vi "GreyRings.vi"(8 "error in (no error)":errorcluster, 11 "MAUI in":refnum<class "MAUI.lvclass">) -> (0 "error out":errorcluster, 3 "MAUI out":refnum<class "MAUI.lvclass">)   [LabVIEW 2016, in "MAUI.lvclass"]
uses:
  MAUI.lvclass
  MAUI.lvclass/MAUI.ctl
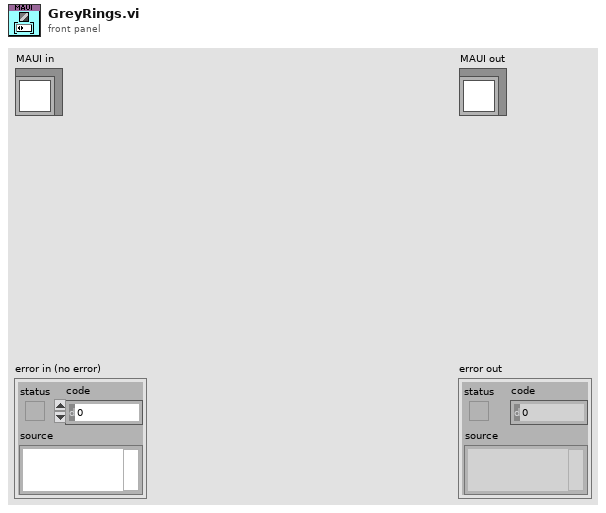
[diagram p1: front panel]
types:
  T1 = typedef "MAUI.lvclass/PanelData.ctl" = cluster{"Subpanel":refnum<vi>, "Ring":refnum<vi>, "Active":i32}
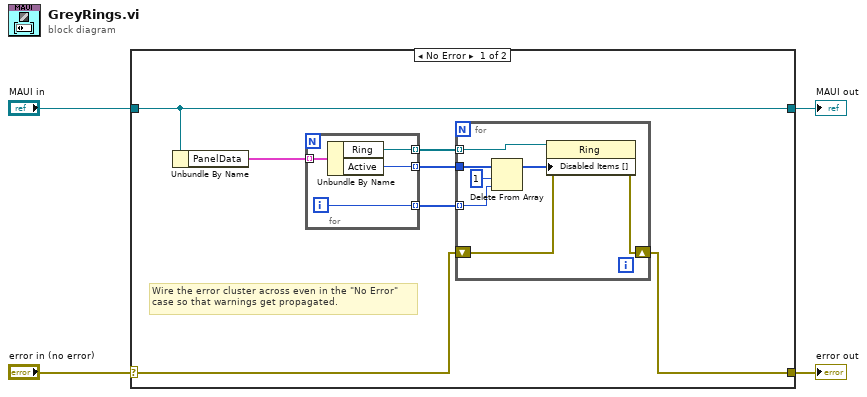
[diagram p0: block diagram]
diagram:
  n1 = case shown="No Error" "error in (no error)" {
    selector: "error in (no error)" -> [w6 w24]
    tunnel: [w5 w24] -> w3
    tunnel: [w11 w23] -> w1
    tunnel: "MAUI in" -> [w11 w23]
    frame No Error {
      # "Wire the error cluster across even in the \"No Error\"\ncase so that warnings get propagated."
      n2 = Unbundle By Name(w11) -> ("PanelData"=w10:T1[])
      n3 = for {
        tunnel: w10 -> [w22] mode=indexing
        tunnel: [w21] -> w9 mode=indexing
        tunnel: [w20] -> w8 mode=indexing
        tunnel: [w19] -> w7 mode=indexing
        i -> [w20]
        n4 = Unbundle By Name(w22) -> ("Ring"=w19:refnum<vi>, "Active"=w21:i32)
      }
      n5 = for {
        tunnel: w9 -> [w17]
        tunnel: w8 -> [w15] mode=indexing
        tunnel: w7 -> [w18] mode=indexing
        shift-right: [w12] -> w5
        shift-left: w6 -> [w13]
        n6 = Delete From Array(array=w17, length=1, index=w15) -> (array with subset deleted=w14:i32[])  [unwired: 1 out]
        n7 = property class="Ring"(reference=w18, error in=w13, "Disabled Items []"=w14) -> (error out=w12:errorcluster)  [unwired: 1 out]
      }
    }
    frame Error {
    }
  }
  "error out" <- w3
  "MAUI out" <- w1
